vi "Compare Unequal Strings.vi"(8 "error in (no error)":errorcluster, 11 "Dummy In":refnum<class "Example Test Case.lvclass">) -> (0 "error out":errorcluster, 3 "Dummy Out":refnum<class "Example Test Case.lvclass">)   [LabVIEW 2020, in "Example Test Case.lvclass"]
doc: "Passing test"
uses:
  Example Test Case.lvclass
  C:/git/astemes-lunit/source/API/LUnit Test Case/LUnit Test Case.lvclass
  API/LUnit Test Case/LUnit Test Case.lvclass/LUnit Test Case.ctl
  455f979b-002d-47f7-b6ef-15e8457416ea.vi
  API/LUnit Test Case/Private/Append Pass Result.vi
  API/LUnit Test Case/Private/Append Fail Result.vi
  455f979b-002d-47f7-b6ef-15e8457416ea.vi/9c5d11cd-9439-4240-a1ee-d9baace9c924.vi
  API/LUnit Test Case/Private/Run In UI.vi
  <vilib>/Utility/error.llb/Clear Errors.vi
  Example Test Case.lvclass/Example Test Case.ctl
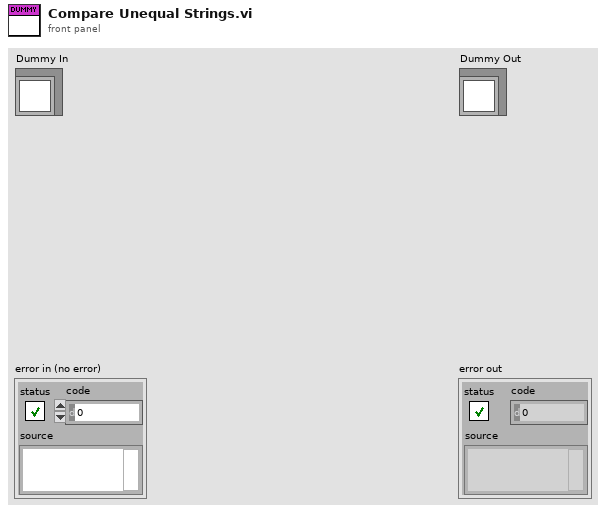
[diagram p1: front panel]
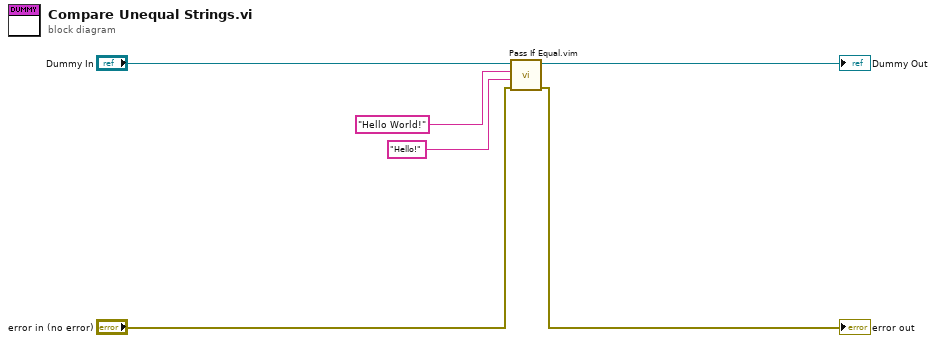
[diagram p0: block diagram]
diagram:
  n1 = call "Pass If Equal.vim"("error in (no error)"="error in (no error)", "Actual"="Hello!" ("Description"), "Expected"="Hello World!" ("Description"), "LUnit Test Case In"="Dummy In") -> ("error out"=→"error out":errorcluster, "LUnit Test Case Out"=→"Dummy Out":refnum<class "Example Test Case.lvclass">)  [unwired: 6 in]
